vi "Target Motor Start and Stop.vi"(7 "Mode":enum16{"Start", "Stop"}(ring), 8 "Error In":errorcluster, 11 "Motion Resource":refnum<k21>="nism://NI-PXIe8880-2F1836AB/AKM74L Motor") -> (0 "Error Out":errorcluster)   [LabVIEW 2018, in "COBRA Kollmorgen Motor IO Library.lvlib"]
uses:
  <vilib>/Motion/Express/_s/nimc.ex.power.power.axis.vi
  <vilib>/Motion/BlockNode/FB.NIMotion.xnode
  COBRA Kollmorgen Motor IO Library.lvlib
  <resource>/objmgr/nimcai.rc
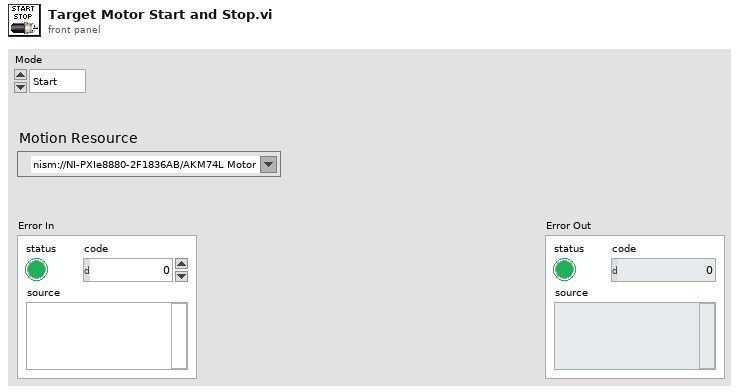
[diagram p1: front panel]
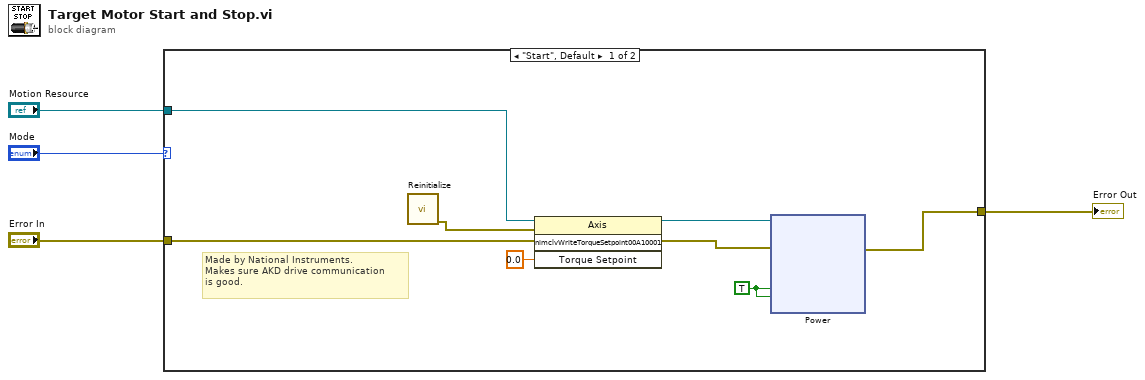
[diagram p0: block diagram]
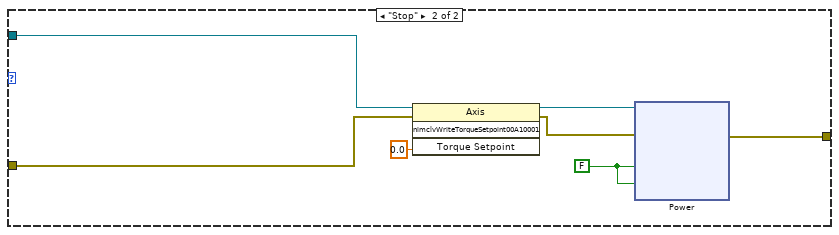
[diagram p2: hidden frame]
diagram:
  n1 = case shown="\"Start\", Default" "Mode" {
    tunnel: "Error In" -> [w9 w25]
    tunnel: [w8 w23] -> w2
    tunnel: "Motion Resource" -> [w5 w22]
    frame "Start", Default {
      w10 = TRUE ("Enable Drive Enable")
      # "Made by National Instruments.\nMakes sure AKD drive communication\nis good."
      n2 = call "Reinitialize.vi"() -> ("error out"=w7:errorcluster)  [unwired: 11 in]
      n3 = invoke on="Invoke Node" class="Axis" method="nimclvWriteTorqueSetpoint00A10001"(reference=w5, error in=w7, "Torque Setpoint"=0.0) -> (reference out=w6:refnum<k21>)  [unwired: 1 in, 3 out]
      n4 = xnode ("Power")("enable axis"=w10, "enable drive"=w10, "resource"=w6, "error in"=w9) -> ("error out"=w8:errorcluster)  [unwired: 1 out]
    }
    frame "Stop" {
      w26 = FALSE ("enable axis")
      n5 = invoke on="Invoke Node" class="Axis" method="nimclvWriteTorqueSetpoint00A10001"(reference=w22, error in=w25, "Torque Setpoint"=0.0) -> (reference out=w28:refnum<k21>, error out=w24:errorcluster)  [unwired: 1 in, 2 out]
      n6 = xnode ("Power")("enable axis"=w26, "enable drive"=w26, "resource"=w28, "error in"=w24) -> ("error out"=w23:errorcluster)  [unwired: 1 out]
    }
  }
  "Error Out" <- w2
